vi "Section Points.vi"(9 "Period":dbl, 10 "Delay":dbl) -> (2 "Seciton Points":u16)   [LabVIEW 2020, in "Actor_AFG.lvlib"]
uses:
  Actor_AFG.lvlib
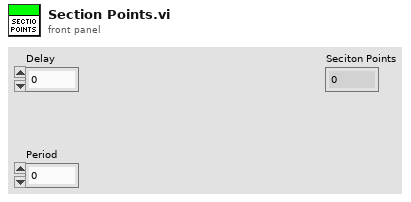
[diagram p1: front panel]
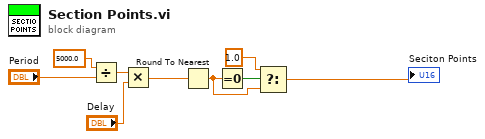
[diagram p0: block diagram]
diagram:
  n1 = Divide(x=5000.0, y="Period") -> (x/y=w8:dbl)
  n2 = Multiply(x=w8, y="Delay") -> (x*y=w5:dbl)
  n3 = Round To Nearest(number=w5) -> (nearest integer value=w2:dbl)
  n4 = Equal To 0?(x=w2) -> (x = 0?=w4:bool)
  n5 = Select(t=1.0, s=w4, f=w2) -> (s? t:f=→"Seciton Points":dbl)
